vi "close.vi"(8 "error in":errorcluster, 11 "shared memory module runtime":refnum<class "Shared Memory Runtime.lvclass">) -> (0 "error out":errorcluster)   [LabVIEW 2013, in "Shared Memory Runtime.lvclass"]
doc: "Provides an interface for terminating a module instance. While this interface performs no operations, a child should close and deallocate any open references or memory.Copyright 2016 National Instruments Corporation\n\nLicensed under the Apache License, Version 2.0 (the \"License\"); you may not use this file except in compliance with the License. You may obtain a copy of the License at http://www.apache.org/licenses/LICENSE-2.0\nUnless required by applicable law or agreed to in writing, software distributed under the License is distributed on an \"AS IS\" BASIS, WITHOUT WARRANTIES OR CONDITIONS OF ANY KIND, either express or implied. See the License for the specific language governing permissions and limitations under the License."
uses:
  Shared Memory Runtime.lvclass
  Shared Memory Runtime.lvclass/Shared Memory Runtime.ctl
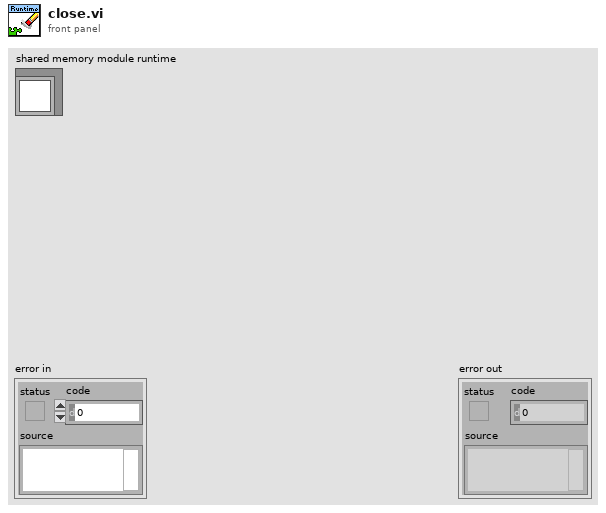
[diagram p1: front panel]
types:
  T1 = typedef "Shared Memory Runtime.lvclass/shared memory module runtime.ctl" = cluster{"refnum":refnum<file>, "name":string, "data type":T2, "number of tags":i32, "indices":cluster{"index":i32[]}, "data array":cluster{"data":dbl[]}, "file array":cluster{"data":dbl[]}}
  T2 = typedef "tag bus.lvlib/tag descriptor.lvclass/Data Type.ctl" = enum16{"Double", "Single", "I64", "I32", "I16", "I8", "U64", "U32", "U16", "U8", "Boolean", "String", "Array of Double", "Array of Single", "Array of I64", "Array of I32", "Array of I16", "Array of I8", "Array of U64", "Array of U32", "Array of U16", "Array of U8", "Array of Boolean", "Array of String"}
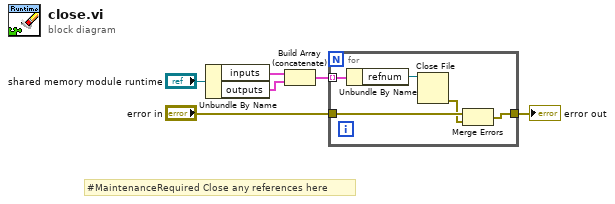
[diagram p0: block diagram]
diagram:
  # "#MaintenanceRequired Close any references here"
  n1 = Unbundle By Name("shared memory module runtime") -> ("inputs"=w5:T1[], "outputs"=w4:T1[])
  n2 = Build Array (concatenate)(w5, w4) -> (w3:T1[])
  n3 = for {
    tunnel: w3 -> [w11] mode=indexing
    tunnel: "error in" -> [w9]
    tunnel: [w7] -> w1
    n4 = Unbundle By Name(w11) -> ("refnum"=w10:refnum<file>)
    n5 = Close File(refnum=w10) -> (error out=w8:errorcluster)  [unwired: 1 in, 1 out]
    n6 = Merge Errors(w9, w8) -> (w7:errorcluster)
  }
  "error out" <- w1
